vi "SetActiveTag__slk_tc.vi"(0 "tree control in":refnum<class "TreeControl.lvclass">, 5 "active tag":string, 11 "error in (no error)":errorcluster) -> (4 "tree control out":refnum<class "TreeControl.lvclass">, 15 "error out":errorcluster)   [LabVIEW 2020, in "TreeControl.lvclass"]
doc: "Sets active tag value."
uses:
  Library/TreeControl.lvclass
  Library/TreeControl.lvclass/TreeControl.ctl
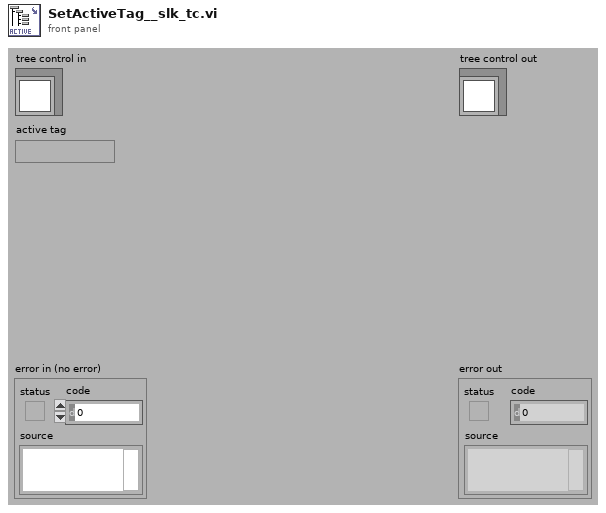
[diagram p1: front panel]
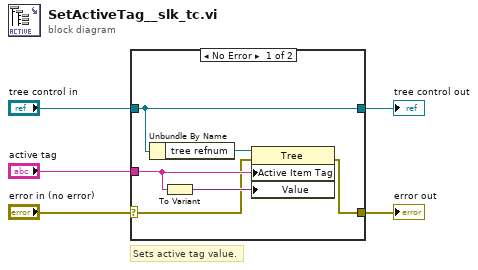
[diagram p0: block diagram]
diagram:
  # "Sets active tag value."
  n1 = case shown="No Error" "error in (no error)" {
    selector: "error in (no error)" -> [w7 w13]
    tunnel: [w6 w13] -> w4
    tunnel: [w11 w12] -> w2
    tunnel: "tree control in" -> [w11 w12]
    tunnel: "active tag" -> [w8 _]
    frame No Error {
      n2 = Unbundle By Name(w11) -> ("tree refnum"=w10:refnum<vi>)
      n3 = To Variant(anything=w8) -> (Variant=w9:variant)
      n4 = property class="Tree"(reference=w10, error in=w7, "Active Item Tag"=w8, "Value"=w9) -> (error out=w6:errorcluster)  [unwired: 1 out]
    }
    frame Error {
    }
  }
  "error out" <- w4
  "tree control out" <- w2
